vi "测量参数设置.vi"(8 "错误输入":errorcluster caption="错误常量") -> (0 "错误输出":errorcluster caption="错误常量")   [LabVIEW 2018]
uses:
  gbl.vi
panel:
  out "路径":path
  in  "取消按钮":bool
  in  "衰减上限":dbl=1.0
  in  "衰减下限":dbl
  in  "声速上限":dbl=1100.0
  in  "声速下限":dbl=900.0
  out "本次监测名称":string
  in  "监测曲线精度":i32=1 min=1 max=100
  in  "确定按钮":bool
  in  "采样间隔/ms":dbl=500.0
  in  "流道间隙/mm":dbl=5.0
  # "测量参数设定"
  # "本次监测名称"
  # "数据保存路径"
  # "<"
  # "<"
  # "材料声速/m/s"
  # "<"
  # "<"
  # "声衰减/dB/m"
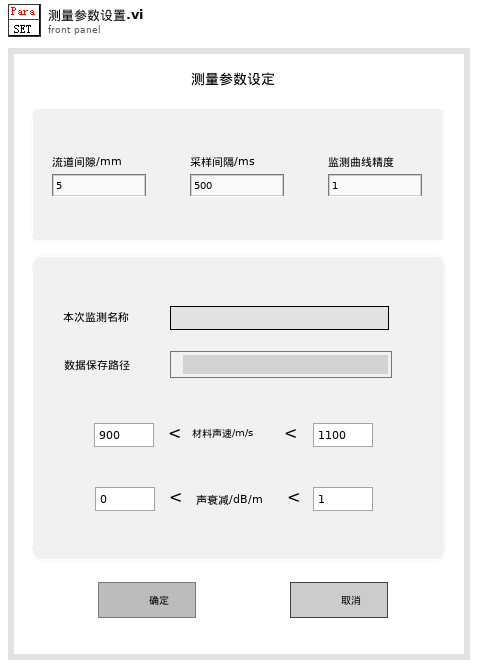
[diagram p1: front panel]
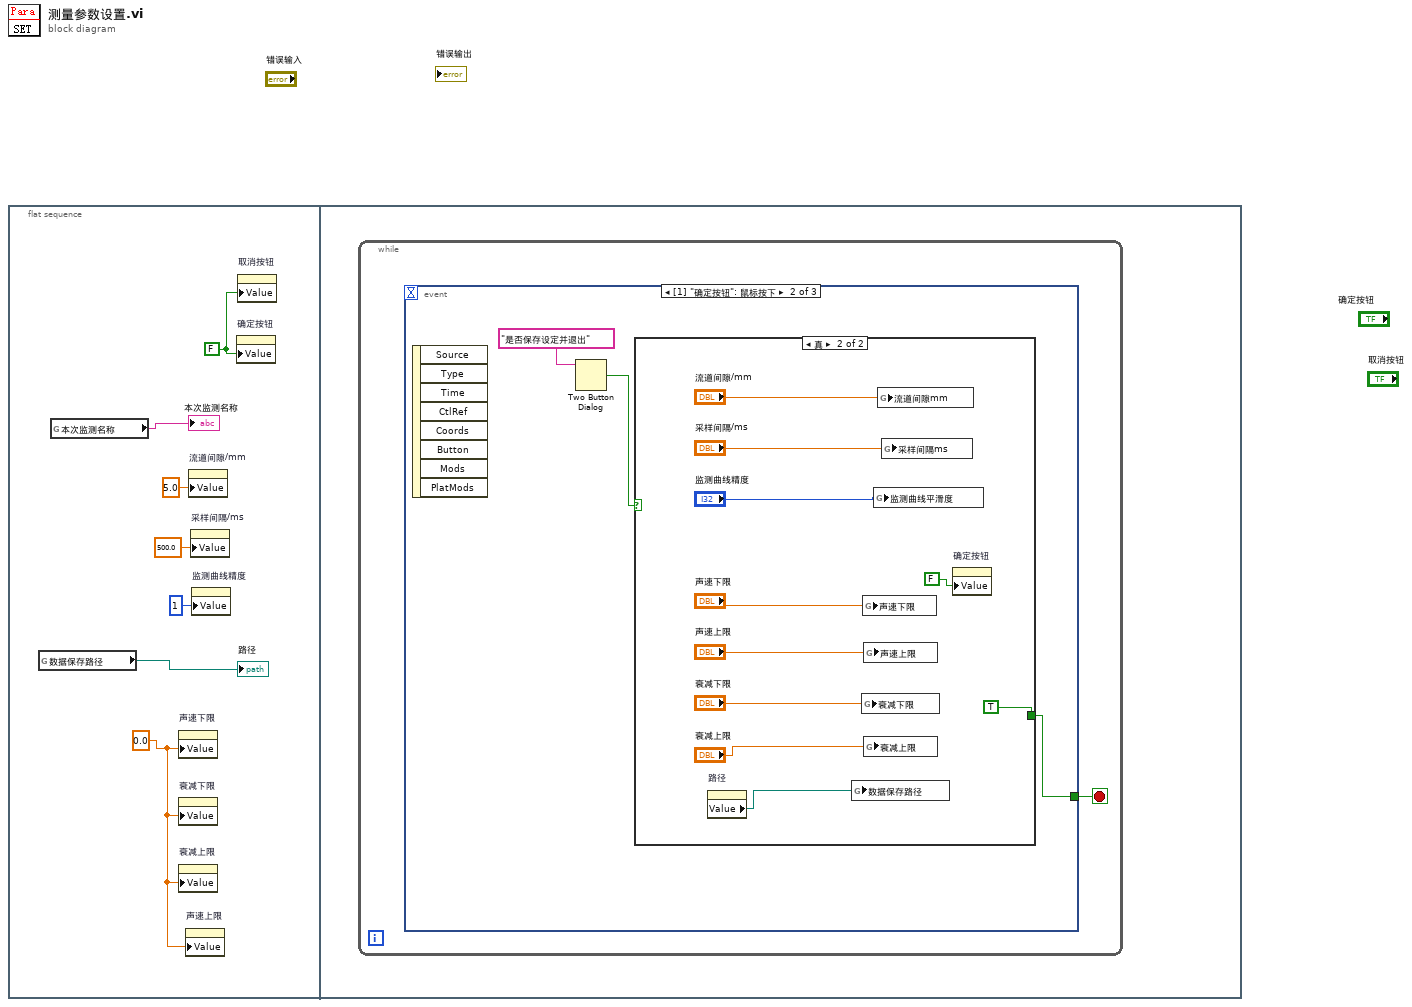
[diagram p0: block diagram]
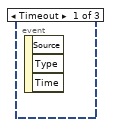
[diagram p2: hidden frame]
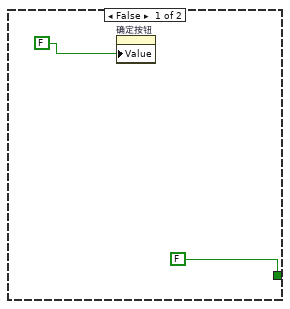
[diagram p3: hidden frame]
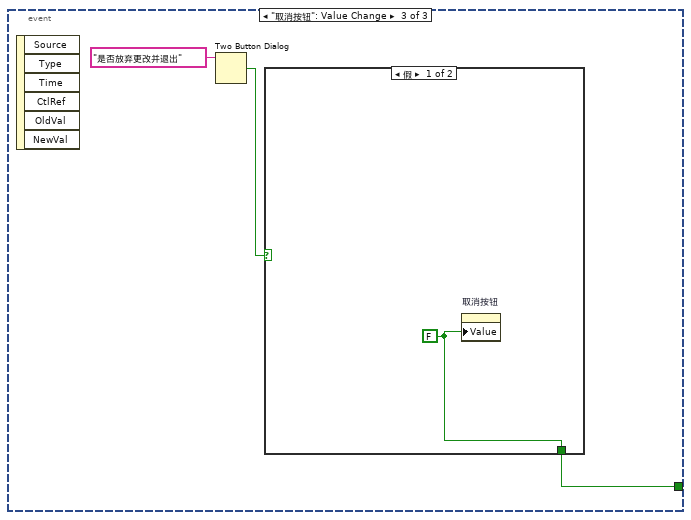
[diagram p4: hidden frame]
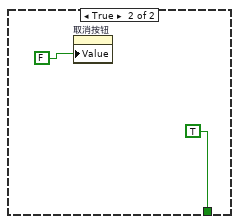
[diagram p5: hidden frame]
diagram:
  n1 = flat-sequence {
    frame #0 {
      w4 = 0.0
      w3 = FALSE ("确定按钮")
      n2 = global read "gbl.vi" "数据保存路径"() -> (→"路径":path)
      n3 = global read "gbl.vi" "本次监测名称"() -> (→"本次监测名称":string)
      n4 = property on="声速下限" class="DigNum (严格)"("Value"=w4) -> ()  [unwired: 2 in, 2 out]
      n5 = property on="衰减下限" class="DigNum (严格)"("Value"=w4) -> ()  [unwired: 2 in, 2 out]
      n6 = property on="衰减上限" class="DigNum (严格)"("Value"=w4) -> ()  [unwired: 2 in, 2 out]
      n7 = property on="声速上限" class="DigNum (严格)"("Value"=w4) -> ()  [unwired: 2 in, 2 out]
      n8 = property on="流道间隙/mm" class="DigNum (严格)"("Value"=5.0 ("流道间隙/mm")) -> ()  [unwired: 2 in, 2 out]
      n9 = property on="采样间隔/ms" class="DigNum (严格)"("Value"=500.0 ("采样间隔/ms")) -> ()  [unwired: 2 in, 2 out]
      n10 = property on="监测曲线精度" class="DigNum (严格)"("Value"=1 ("监测曲线精度")) -> ()  [unwired: 2 in, 2 out]
      n11 = property on="确定按钮" class="Bool (严格)"("Value"=w3) -> ()  [unwired: 2 in, 2 out]
      n12 = property on="取消按钮" class="Bool (严格)"("Value"=w3) -> ()  [unwired: 2 in, 2 out]
    }
    frame #1 {
      n13 = while {
        stop <- w8 stop-if-true
        n14 = event shown="[1] \"确定按钮\": 鼠标按下" {
          selector: _ -> [_ _ _]
          dyn-events: _ -> [_ _ _]
          timeout: _ -> [_ _ _]
          tunnel: [_ w9 w24] -> w8
          event Timeout {
            n15 = event-data() -> ()  [unwired: 1 in, 3 out]
          }
          event "确定按钮": Mouse Down {
            n16 = event-data() -> ()  [unwired: 1 in, 8 out]
            n17 = Two Button Dialog(message="是否保存设定并退出" ("消息")) -> (T button?=w10:bool)  [unwired: 2 in]
            n18 = case shown="真" w10 {
              tunnel: [FALSE TRUE] -> w9
              frame False {
                n19 = property on="确定按钮" class="Bool (严格)"("Value"=FALSE) -> ()  [unwired: 2 in, 2 out]
              }
              frame True {
                n20 = property on="路径" class="Path"() -> ("Value"=w14:path)  [unwired: 2 in, 2 out]
                n21 = global write "gbl.vi" "数据保存路径"(w14) -> ()
                n22 = global write "gbl.vi" "衰减下限"("衰减下限") -> ()
                n23 = global write "gbl.vi" "声速下限"("声速下限") -> ()
                n24 = global write "gbl.vi" "声速上限"("声速上限") -> ()
                n25 = global write "gbl.vi" "衰减上限"("衰减上限") -> ()
                n26 = global write "gbl.vi" "监测曲线平滑度"("监测曲线精度") -> ()
                n27 = global write "gbl.vi" "流道间隙mm"("流道间隙/mm") -> ()
                n28 = global write "gbl.vi" "采样间隔ms"("采样间隔/ms") -> ()
                n29 = property on="确定按钮" class="Bool (严格)"("Value"=FALSE) -> ()  [unwired: 2 in, 2 out]
              }
            }
          }
          event "取消按钮": Value Change {
            n30 = event-data() -> ()  [unwired: 1 in, 6 out]
            n31 = Two Button Dialog(message="是否放弃更改并退出" ("消息")) -> (T button?=w25:bool)  [unwired: 2 in]
            n32 = case shown="假" w25 {
              tunnel: [w27 TRUE] -> w24
              frame False {
                w27 = FALSE
                n33 = property on="取消按钮" class="Bool (严格)"("Value"=w27) -> ()  [unwired: 2 in, 2 out]
              }
              frame True {
                n34 = property on="取消按钮" class="Bool (严格)"("Value"=FALSE) -> ()  [unwired: 2 in, 2 out]
              }
            }
          }
        }
      }
    }
  }
